vi "InitHardware.vi"(8 "error in (no error)":errorcluster, 11 "Point Grey Camera in":refnum<class "Point Grey Camera.lvclass">) -> (0 "error out":errorcluster, 1 "bit depth":string, 2 "Image Type":T1 items=["Grayscale (U8)", "Grayscale (I16)", "Grayscale (SGL)", "Complex (CSG)", "RGB (U32)", "HSL (U32)", "RGB (U64)", "Grayscale (U16)"], 3 "Point Grey Camera out":refnum<class "Point Grey Camera.lvclass">)   [LabVIEW 2020, in "Point Grey Camera.lvclass"]
uses:
  Point Grey Camera.lvclass
  Point Grey Camera.lvclass/Point Grey Camera.ctl
  <vilib>/vision/driver/NI_Vision_Acquisition_Software.lvlib
  <resource>/objmgr/imaqdx.rc
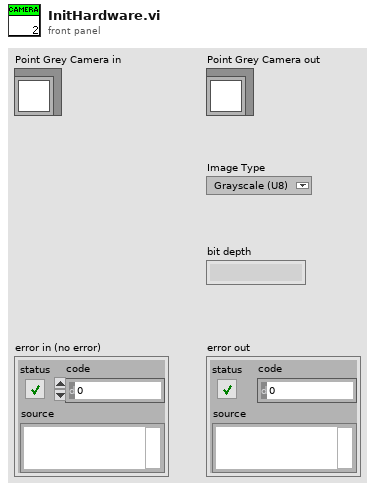
[diagram p1: front panel]
types:
  T1 = typedef "Image Type" = u32
  T2 = typedef "OnOffTypeDef.ctl" = enum16{"off", "on"}
  T3 = typedef "TriggerModeString_TypDEf.ctl" = cluster{"On":string, "Off":string}
  T4 = typedef "CamAtributes_TypDEf.ctl" = cluster{"Gain":string, "Shutter":string, "TriggerDelay":string, "TriggerMode":string, "ROI Width":string, "ROI Height":string, "ROI OffsetX":string, "ROI OffsetY":string, "TriggerSource":string}
  T5 = typedef "IMAQdx.ctl" = refnum<k21>
  T6 = typedef "TriggerSource_TypDEF.ctl" = cluster{"Software":string, "External":string, "Execute":string}
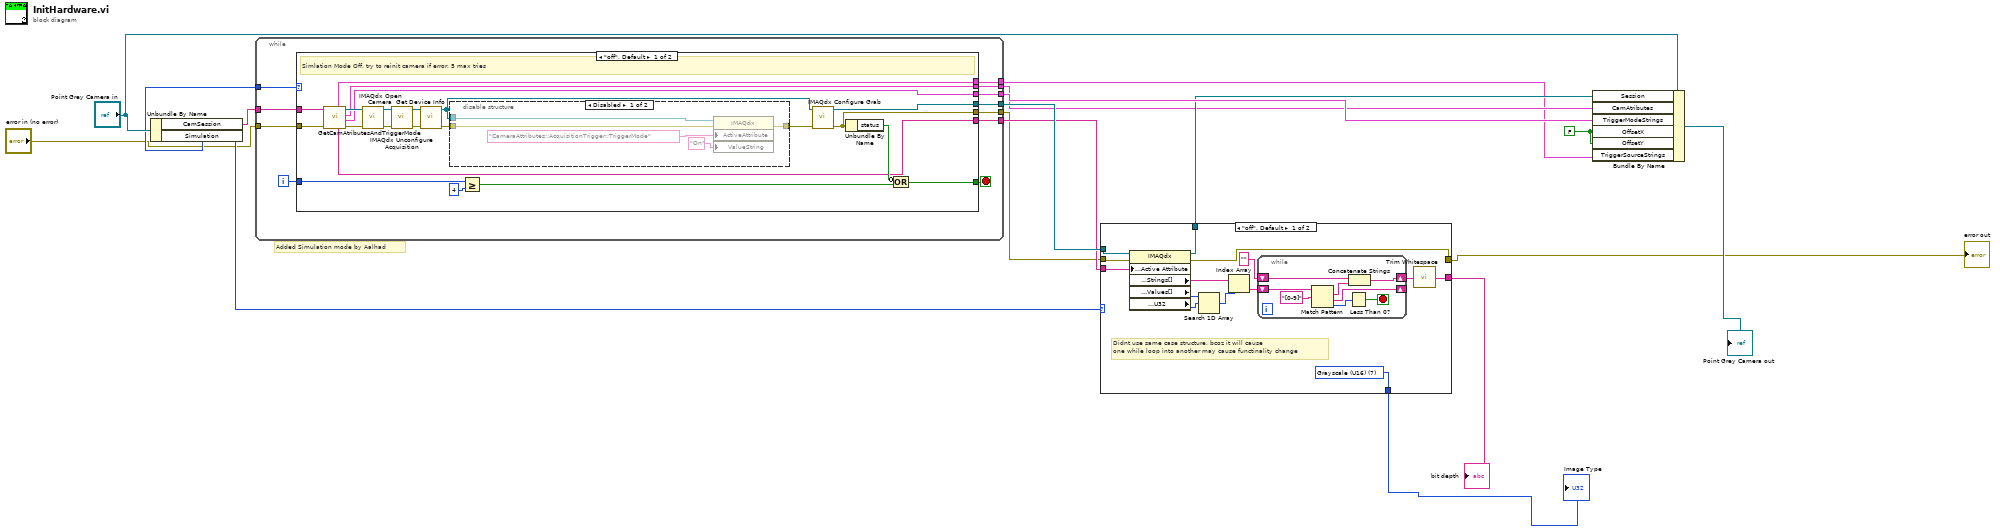
[diagram p0: block diagram]
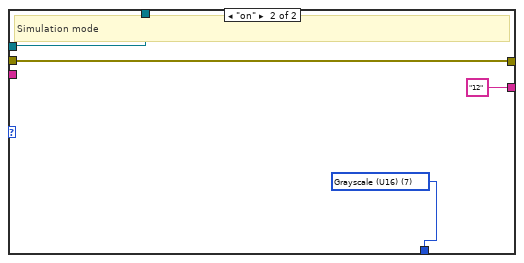
[diagram p2: hidden frame]
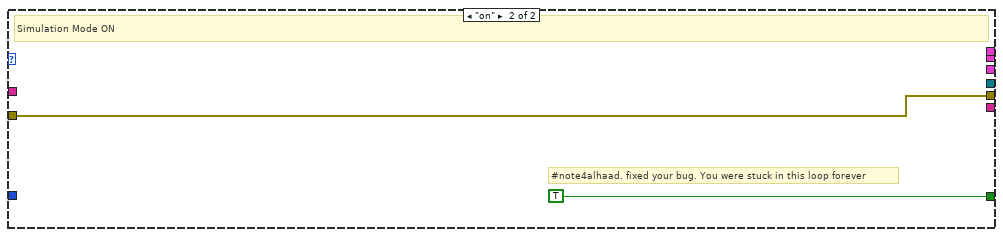
[diagram p4: hidden frame]
diagram:
  w4 = FALSE ("OffsetX")
  # "Added Simulation mode by Aalhad"
  n1 = Unbundle By Name("Point Grey Camera in") -> ("CamSession"=w3:string, "Simulation"=w10:T2)
  n2 = while "try to reinit camera if error. 5 max tries" {
    tunnel: [w27] -> w2
    tunnel: [w26] -> w11
    tunnel: "error in (no error)" -> [w25]
    tunnel: w3 -> [w24]
    tunnel: [w22] -> w5
    tunnel: [w20] -> w9
    tunnel: w10 -> [w19]
    tunnel: [w18] -> w12
    tunnel: [w17] -> w1
    i -> [w23]
    stop <- w21 stop-if-true
    n3 = case shown="\"off\", Default" w19 {
      tunnel: [w29 _] -> w18
      tunnel: [w47 _] -> w27
      tunnel: [w46 _] -> w26
      tunnel: w25 -> [w45 w57]
      tunnel: w24 -> [w43 _]
      tunnel: w23 -> [w41 _]
      tunnel: [w39 w57] -> w22
      tunnel: [w36 TRUE] -> w21
      tunnel: [w35 _] -> w20
      tunnel: [w28 _] -> w17
      frame "off", Default {
        # "Simlation Mode Off, try to reinit camera if error. 5 max tries"
        n4 = call "GetCamAtributesAndTriggerMode.vi"("error in"=w45, "IMAQdx Session"=w43) -> ("error out"=w44:errorcluster, "TriggerModeStrings"=w46:T3, "CamAtributes"=w47:T4, "IMAQdx Session 2"=w48:T5, "PixelFormat"=w35:string, "TriggerSourceStrings"=w28:T6)  [unwired: 4 in]
        n5 = call <vilib>:"IMAQdx Open Camera.vi"("error in"=w44, "Session In"=w48) -> ("error out"=w49:errorcluster, "Session Out"=w42:T5)  [unwired: 1 in, 7 out]
        n6 = call <vilib>:"IMAQdx Unconfigure Acquisition.vi"("error in"=w49, "Session In"=w42) -> ("error out"=w32:errorcluster, "Session Out"=w33:T5)  [unwired: 8 out]
        n7 = call "Get Device Info.vi"("error in (no error)"=w32, "image in"=w33) -> ("error out"=w30:errorcluster, "image out"=w31:T5)  [unwired: 8 in]
        n8 = disable-structure shown="Disabled" {
          disable-tunnel: w31 -> [w52 _]
          disable-tunnel: w30 -> [w51 w55]
          disable-tunnel: [w50 w55] -> w34
          frame Disabled {
            n9 = property class="IMAQdx"(reference=w52, error in=w51, "ActiveAttribute"="CameraAttributes::AcquisitionTrigger::TriggerMode", "ValueString"="On") -> (error out=w50:errorcluster)  [unwired: 1 out]
          }
          frame Enabled {
          }
        }
        n10 = Greater Or Equal?(x=w41, y=4) -> (x >= y?=w37:bool)
        n11 = call <vilib>:"IMAQdx Configure Grab.vi"("error in"=w34, "Session In"=w31) -> ("error out"=w39:errorcluster, "Session Out"=w29:T5)  [unwired: 1 in, 7 out]
        n12 = Unbundle By Name(w39) -> ("status"=w38:bool)
        n13 = Compound Arithmetic op=OR(invert w38, w37) -> (w36:bool)
      }
      frame "on" {
        # "#note4alhaad. fixed your bug. You were stuck in this loop forever"
        # "Simulation Mode ON"
      }
    }
  }
  n14 = case shown="\"off\", Default" w10 {
    tunnel: w5 -> [w64 w81]
    tunnel: [w63 w82] -> w6
    tunnel: [w62 w81] -> w13
    tunnel: [w61 "12" ("trimmed string")] -> w8
    tunnel: w9 -> [w60 _]
    tunnel: w12 -> [w59 w82]
    tunnel: [w58 w80] -> w14
    frame "off", Default {
      w58 = T1 7 items=["Grayscale (U8)", "Grayscale (I16)", "Grayscale (SGL)", "Complex (CSG)", "RGB (U32)", "HSL (U32)", "RGB (U64)", "Grayscale (U16)"] ("Image Type")
      # "Didnt use same case structure, bcoz it will cause \none while loop into another may cause functinality change"
      n15 = property class="IMAQdx"(reference=w59, error in=w64, "Camera Attributes:Active Attribute"=w60) -> (reference out=w63:T5, error out=w62:errorcluster, "Camera Attributes:Enum:Strings[]"=w67:string[], "Camera Attributes:Enum:Values[]"=w65:u32[], "Camera Attributes:Value:U32"=w66:u32)
      n16 = Search 1D Array(1D array=w65, element=w66) -> (index of element=w68:i32)  [unwired: 1 in]
      n17 = Index Array(array=w67, index=w68) -> (element=w69:string)
      n18 = while {
        shift-right: [w77] -> _
        shift-left: w69 -> [w79]
        shift-right: [w73] -> w71
        shift-left: "" -> [w74]
        stop <- w75 stop-if-true
        n19 = Match Pattern(string=w79, regular expression="[0-9]") -> (match substring=w72:string, after substring=w77:string, offset past match=w76:i32)  [unwired: 1 in, 1 out]
        n20 = Less Than 0?(x=w76) -> (x < 0?=w75:bool)
        n21 = Concatenate Strings(w74, w72) -> (w73:string)
      }
      n22 = call <vilib>:"Trim Whitespace.vi"("string"=w71) -> ("trimmed string"=w61:string)  [unwired: 1 in]
    }
    frame "on" {
      w80 = T1 7 items=["Grayscale (U8)", "Grayscale (I16)", "Grayscale (SGL)", "Complex (CSG)", "RGB (U32)", "HSL (U32)", "RGB (U64)", "Grayscale (U16)"] ("Image Type")
      # "Simulation mode"
    }
  }
  "Image Type" <- w14
  "error out" <- w13
  "bit depth" <- w8
  n23 = Bundle By Name(cluster="Point Grey Camera in", "Session"=w6, "CamAtributes"=w2, "TriggerModeStrings"=w11, "OffsetX"=w4, "OffsetY"=w4, "TriggerSourceStrings"=w1) -> (→"Point Grey Camera out":refnum<class "Point Grey Camera.lvclass">)
